vi "Override input Value.vi"(5 "Starting Override Value (0-1)":dbl, 7 "Min Value To Overide (0-1)":dbl, 10 "OverRide Value (0-1)":T1 scale=-1.0..1.0 scale format="%.1f", 11 "Value In (0-1)":T1 scale=-1.0..1.0 scale format="%.1f") -> (3 "Value Out":T1 scale=-1.0..1.0 scale format="%.1f")   [LabVIEW 2023]
uses:
  Shared Code/TypeDefs/Level_Velocity plus-minus 1.ctl
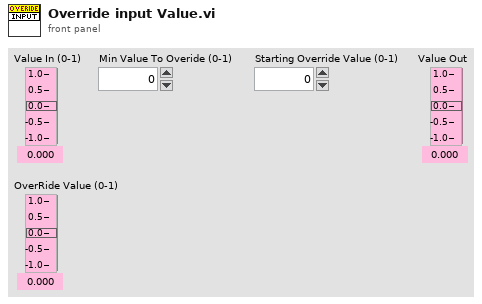
[diagram p1: front panel]
types:
  T1 = typedef "Level_Velocity plus-minus 1.ctl" = dbl
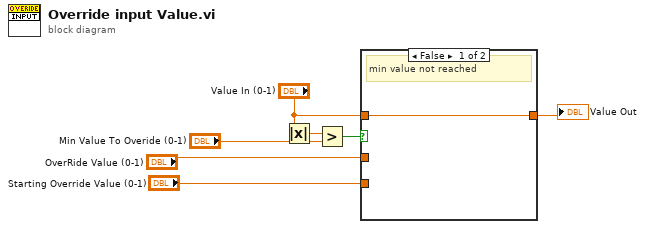
[diagram p0: block diagram]
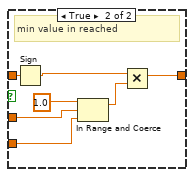
[diagram p2: hidden frame]
diagram:
  n1 = Absolute Value(x="Value In (0-1)") -> (abs(x)=w3:T1)
  n2 = Greater?(x=w3, y="Min Value To Overide (0-1)") -> (0:w5:bool)
  n3 = case shown="False" w5 {
    tunnel: "Value In (0-1)" -> [w8 w15]
    tunnel: [w8 w14] -> w7
    tunnel: "OverRide Value (0-1)" -> [_ w12]
    tunnel: "Starting Override Value (0-1)" -> [_ w9]
    frame False {
      # "min value not reached"
    }
    frame True {
      # "min value in reached"
      n4 = Sign(1:w15) -> (0:w10:T1)
      n5 = In Range and Coerce(upper limit=T1 1.0 ("lower limit"), x=w12, lower limit=w9) -> (coerced(x)=w11:T1)  [unwired: 1 out]
      n6 = Multiply(x=w10, y=w11) -> (x*y=w14:T1)
    }
  }
  "Value Out" <- w7
